vi "Run.vi"(9 "Team in":refnum<class "Team.lvclass">, 11 "MySquare in":refnum<class "MySquare.lvclass">) -> (1 "Team out":refnum<class "Team.lvclass">, 2 "Run Result":T1, 3 "Square out":refnum<class "Square.lvclass">)   [LabVIEW 2020, in "Rain.lvlib" / "MySquare.lvclass"]
doc: "This VI is called on every active square each turn of the game for the square to decide what action to take."
uses:
  MySquare.lvclass
  C:/dev/lv20CE/sol-squarebattle/ProjectTemplates/Source/SummerOfLabVIEW/SquareBattle/template/SquareBattle/Square/Square.lvclass
  SquareBattle/Square/Square.lvclass
  SquareBattle/Run Result.ctl
  SquareBattle/Action.ctl
  SquareBattle/Direction.ctl
  SquareBattle/Team/Team.lvclass
  SquareBattle/Square/Square.lvclass/Square.ctl
  SquareBattle/SquareBattle.lvlib
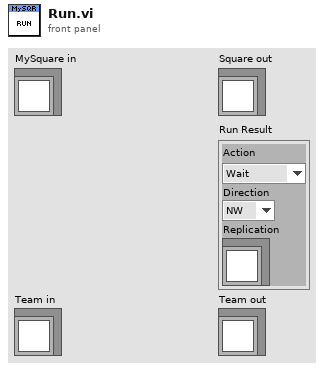
[diagram p1: front panel]
types:
  T1 = typedef "SquareBattle.lvlib/Run Result.ctl" = cluster{"Action":T2, "Direction":T3, "Replication":refnum<class "Square.lvclass">}
  T2 = typedef "SquareBattle.lvlib/Action.ctl" = enum16{"Wait", "Move", "Attack", "Replicate"}
  T3 = typedef "SquareBattle.lvlib/Direction.ctl" = enum16{"NW", "N", "NE", "E", "SE", "S", "SW", "W"}
  T4 = typedef "SquareBattle.lvlib/Location Status.ctl" = cluster{"Empty":bool, "Friend":bool, "Enemy":bool}
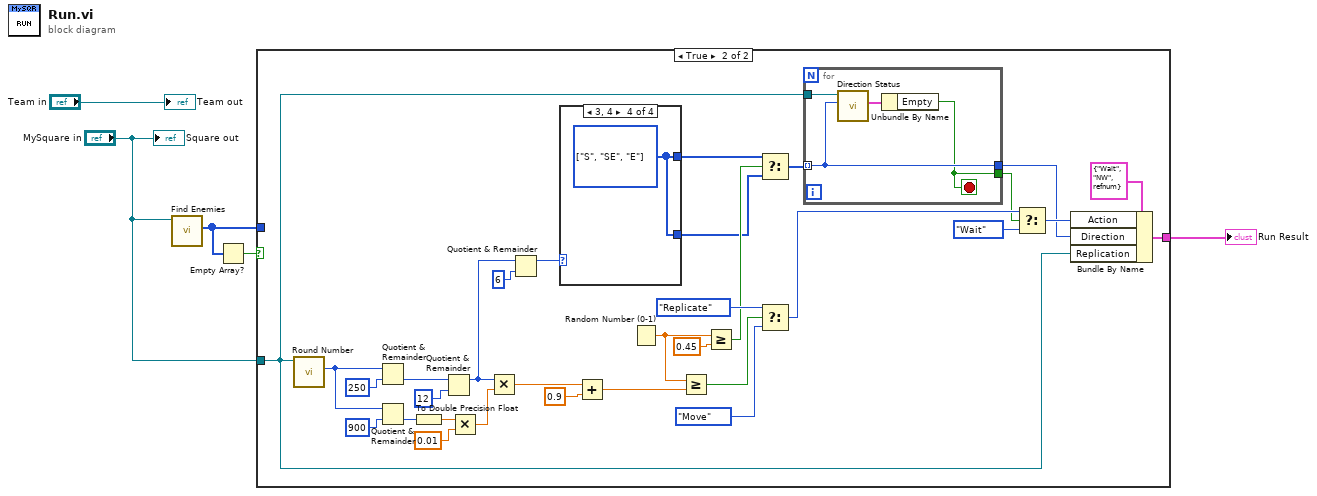
[diagram p0: block diagram]
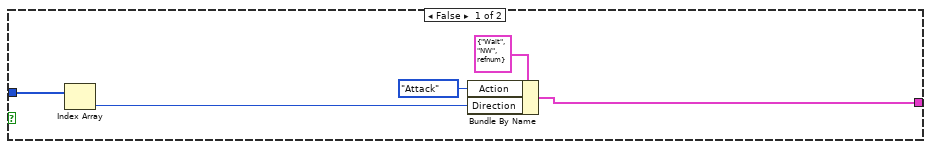
[diagram p2: hidden frame]
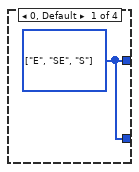
[diagram p3: hidden frame]
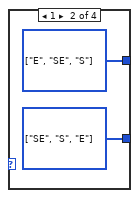
[diagram p4: hidden frame]
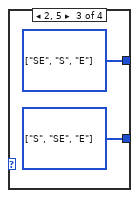
[diagram p5: hidden frame]
diagram:
  n1 = call "Find Enemies.vi"("Square"="MySquare in") -> ("Enemy Directions"=w2:T3[])  [unwired: 10 in]
  n2 = Empty Array?(array=w2) -> (empty?=w1:bool)
  n3 = case shown="True" w1 {
    tunnel: [w9 w15] -> w4
    tunnel: w2 -> [w8 _]
    tunnel: "MySquare in" -> [_ w13]
    frame False {
      n4 = Index Array(array=w8) -> (element=w7:T3)  [unwired: 1 in]
      n5 = Bundle By Name(cluster=T1 {"Action"=enum."Wait", "Direction"=enum."NW", "Replication"=refnum} ("Run Result"), "Action"=Action."Attack", "Direction"=w7) -> (w9:T1)
    }
    frame True {
      n6 = call "Round Number.vi"("Square in"=w13) -> ("Round Number"=w17:u32)  [unwired: 10 in]
      n7 = Quotient & Remainder(x=w17, y=u32 250) -> (floor(x/y)=w29:u32)  [unwired: 1 out]
      n8 = Quotient & Remainder(x=w17, y=u32 900) -> (floor(x/y)=w20:u32)  [unwired: 1 out]
      n9 = To Double Precision Float(number=w20) -> (double precision float=w11:dbl)
      n10 = Quotient & Remainder(x=w29, y=u32 12) -> (x-y*floor(x/y)=w23:u32)  [unwired: 1 out]
      n11 = Multiply(x=w11, y=0.01) -> (x*y=w18:dbl)
      n12 = Multiply(x=w23, y=w18) -> (x*y=w28:dbl)
      n13 = Quotient & Remainder(x=w23, y=u32 6) -> (x-y*floor(x/y)=w22:u32)  [unwired: 1 out]
      n14 = case shown="3, 4" w22 {
        tunnel: [w43 w45 w47 w48] -> w33
        tunnel: [w43 w44 w46 w48] -> w34
        frame 0, Default {
          w43 = T3[] [enum."E", enum."SE", enum."S"] items=["NW", "N", "NE", "E", "SE", "S", "SW", "W"]
        }
        frame 1 {
          w44 = T3[] [enum."SE", enum."S", enum."E"] items=["NW", "N", "NE", "E", "SE", "S", "SW", "W"]
          w45 = T3[] [enum."E", enum."SE", enum."S"] items=["NW", "N", "NE", "E", "SE", "S", "SW", "W"]
        }
        frame 2, 5 {
          w46 = T3[] [enum."S", enum."SE", enum."E"] items=["NW", "N", "NE", "E", "SE", "S", "SW", "W"]
          w47 = T3[] [enum."SE", enum."S", enum."E"] items=["NW", "N", "NE", "E", "SE", "S", "SW", "W"]
        }
        frame 3, 4 {
          w48 = T3[] [enum."S", enum."SE", enum."E"] items=["NW", "N", "NE", "E", "SE", "S", "SW", "W"]
        }
      }
      n15 = Add(x=w28, y=0.9) -> (x+y=w26:dbl)
      n16 = Random Number (0-1)() -> (number: 0 to 1=w31:dbl)
      n17 = Greater Or Equal?(x=w31, y=w26) -> (x >= y?=w37:bool)
      n18 = Greater Or Equal?(x=w31, y=0.45) -> (x >= y?=w35:bool)
      n19 = Select(t=w33, s=w35, f=w34) -> (s? t:f=w32:T3[])
      n20 = Select(t=Action."Replicate" ("Action"), s=w37, f=Action."Move" ("Action")) -> (s? t:f=w40:T2)
      n21 = for {
        tunnel: [w49] -> w39
        tunnel: w32 -> [w51] mode=indexing
        tunnel: [w51] -> w12
        tunnel: w13 -> [w52]
        stop <- w49 stop-if-true
        n22 = call "Direction Status.vi"("Direction"=w51, "Square"=w52) -> ("Status"=w50:T4)  [unwired: 8 in, 1 out]
        n23 = Unbundle By Name(w50) -> ("Empty"=w49:bool)
      }
      n24 = Select(t=w40, s=w39, f=Action."Wait" ("Action")) -> (s? t:f=w14:T2)
      n25 = Bundle By Name(cluster=T1 {"Action"=enum."Wait", "Direction"=enum."NW", "Replication"=refnum} ("Run Result"), "Action"=w14, "Direction"=w12, "Replication"=w13) -> (w15:T1)
    }
  }
  "Run Result" <- w4
  "Square out" <- "MySquare in"
  "Team out" <- "Team in"
